vi "ConvertCompsNew10.vi"(1 "components 1.2":T2[](array[typedef]) {"component type" items=["standard", "hidden", "system", "unknown", "startup", "image"]}) -> (0 "components 1.0":T1[](array[typedef]))   [LabVIEW 2014]
uses:
  Software 1.2.ctl
  Component Type.ctl
  Software.ctl
  nisyscfg.lvlib
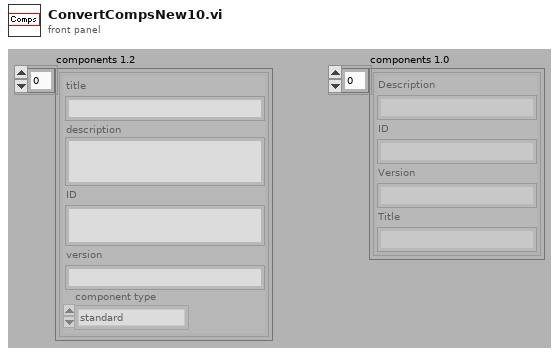
[diagram p1: front panel]
types:
  T1 = typedef "nisyscfg.lvlib/Software.ctl" = cluster{"Description":string, "ID":string, "Version":string, "Title":string}
  T2 = typedef "nisyscfg.lvlib/Software 1.2.ctl" = cluster{"title":string, "description":string, "ID":string, "version":string, "component type":T3}
  T3 = typedef "nisyscfg.lvlib/Component Type.ctl" = u32
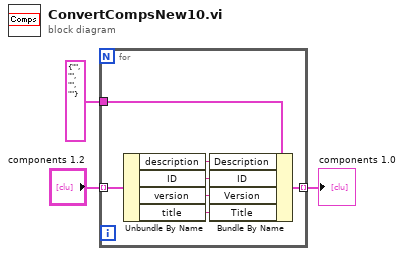
[diagram p0: block diagram]
diagram:
  n1 = for {
    tunnel: "components 1.2" -> [w10] mode=indexing
    tunnel: T1 {"Description"="", "ID"="", "Version"="", "Title"=""} ("Software") -> [w9]
    tunnel: [w8] -> w1 mode=indexing
    n2 = Unbundle By Name(w10) -> ("description"=w7:string, "ID"=w6:string, "version"=w5:string, "title"=w4:string)
    n3 = Bundle By Name(cluster=w9, "Description"=w7, "ID"=w6, "Version"=w5, "Title"=w4) -> (w8:T1)
  }
  "components 1.0" <- w1
